vi "Update FOV.vi"(8 "error in (no error)":errorcluster, 11 "UI ctrl refs":T1) -> (0 "error out":errorcluster)   [LabVIEW 2020]
uses:
  Typedefs/UI ctrl refs cluster.ctl
  Typedefs/Laser control knob.ctl
  Typedefs/Frame Size.ctl
  Typedefs/Plane Mode.ctl
  Typedefs/PMT control knob.ctl
  Typedefs/XY Stage_Move.ctl
  Typedefs/test_fpga_control.ctl
  Acquisition/Typedefs/Ref DAQ Param.ctl
  Experiment Type.ctl
  Biology Information.ctl
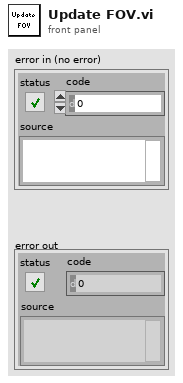
[diagram p1: front panel]
types:
  T1 = typedef "UI ctrl refs cluster.ctl" = cluster{"Top level VI path":path, "Top level VI ref":refnum<vi>, "User menu ref":refnum<k9>, "Sub Panel control":refnum<vi>, "Imaging Param Tab":refnum<vi>, "Occurrence-Start drivers":refnum<k4>, "Occurrence-Speed logging initialised":refnum<k4>, "Occurrence-XYZ stage initialised":refnum<k4>, "Exit button":refnum<vi>, "Status ind":refnum<vi>, "Set as origin":refnum<vi>, "Speed Logging":refnum<vi>, "Time Lapse":refnum<vi>, "Live Imaging":refnum<vi>, "AOL Z Stack":refnum<vi>, "Motor Z Stack":refnum<vi>, "Funct Acq button":refnum<vi>, "Hard Shutter":refnum<vi>, "Virtual Shutter":refnum<vi>, "Laser Power":refnum<vi>, "AOL Mode":refnum<vi>, "Frame Size":refnum<vi>, "Field of View":refnum<vi>, "Dwell Time":refnum<vi>, "Zoom":refnum<vi>, "AOL Z":refnum<vi>, "Objective":refnum<vi>, "Axis":refnum<vi>, "Paths & Names":refnum<vi>, "Experiment folder path (ind.)":refnum<vi>, "Last State (Ind.)":refnum<vi>, "Averages":refnum<vi>, "Angle (degrees)":refnum<vi>, "X centre":refnum<vi>, "Y centre":refnum<vi>, "Plane Mode":refnum<vi>, "# Planes":refnum<vi>, "Z Start":refnum<vi>, "Z Stop":refnum<vi>, "Z Step":refnum<vi>, "PMT 1":refnum<vi>, "PMT 2":refnum<vi>, "Stage XYZ Position":refnum<vi>, "Pockels@Z Start":refnum<vi>, "Pockels@Z Stop":refnum<vi>, "Obtain Z Start":refnum<vi>, "Obtain Z Stop":refnum<vi>, "Live stim.trig.period":refnum<vi>, "Live stim.trig.enable":refnum<vi>, "Movement Correction":refnum<vi>, "Load Reference Image":refnum<vi>, "XY Stage Move":refnum<vi>, "MovCor Cluster":refnum<vi>, "RefDAQParam":refnum<vi>, "Funct. Acq. Pockels Modulation":refnum<vi>, "Ref Laser Power":refnum<vi>, "Enable Video Recording":refnum<vi>, "Video Record-Live Imaging":refnum<vi>, "Video Record-Funct acq":refnum<vi>, "Reference Source":refnum<vi>, "AOL Z-stack Chirps Ready (ind)":refnum<vi>, "Target time between mov.cor. ref triggers (ms)":refnum<vi>, "Funct. Acq. Ref frame save":refnum<vi>, "Tracking button":refnum<vi>, "Show ref plots window":refnum<vi>, "Center freq ind (nm)":refnum<vi>, "Pickup mode (ind)":refnum<vi>, "Logging queue (ind)":refnum<vi>, "Back aperture power (ind.)":refnum<vi>, "Power after objective (ind.)":refnum<vi>, "Switch user":refnum<vi>, "Ls1 Conn. Status":refnum<vi>, "Ls1Tuning Status":refnum<vi>, "Ls1 Faults":refnum<vi>, "Ls1 Connection":refnum<vi>, "Ls1 Mode":refnum<vi>, "Ls1 POWER [mW]":refnum<vi>, "Ls1Shutter":refnum<vi>, "Ls1 Wavelength":refnum<vi>, "Ls1 Note":refnum<vi>, "Ls1 Confirm Wav":refnum<vi>, "Ls1 PreChrp Prism1":refnum<vi>, "Ls1 PreChrp Prism2":refnum<vi>, "Ls1 wav top Ind":refnum<vi>, "Ls1 power top Ind":refnum<vi>, "Ls1 Pump peak Hold":refnum<vi>, "Ls1 Status Ind":refnum<vi>, "Ls1 wav cancel":refnum<vi>, "Experiment Type":refnum<vi>, "Biology Information":refnum<vi>, "Camera recording status":refnum<vi>, "Optimise Obj. Pos.":refnum<vi>}
  T2 = typedef "AOL_Globals.ctl" = cluster{"Imaging Protocol":T3, "Number of POI":u16, "Number of Miniscans":u16, "Number of Trials":u16, "Number of Cycles ":u64, "# Averaged Frames":u16, "Laser power (%)":u8, "Pockels (V)":dbl, "Acquisition Length (sec)":dbl, "Fill time (us)":dbl, "POI Dwell time (us)":dbl, "Miniscan Dwell time per pixel (us)":dbl, "PMT 1":dbl, "PMT 2":dbl, "Back Apperture (mA)":dbl, "Frame Size":T4, "Center Frequency":dbl, "Field of View (um)":dbl, "Field of View (norm)":dbl, "DwellTime (us)":dbl, "Ref Dwell Time (us)":dbl, "Wavelength (nm)":dbl, "Zoom":dbl, "AOL Z":dbl, "AOL Mode":T5, "GridXY":dbl, "GridZ":dbl, "TriggerPeriod (sec)":dbl, "Number of Pixels in Miniscan":u16, "Experiment folder path":path, "X centre":dbl, "Y centre":dbl, "Angle (degrees)":dbl, "Angle Xs (degrees)":dbl, "Angle Ys (degrees)":dbl, "Plane Mode":T6, "Threshold":u16[], "Regenerate Chirps":bool, "Rectangle ROI length (pixels)":u16, "Rectangle ROI height (pixels)":u16, "AOD fill":u16, "StartupDelay":i32, "Samples Wait after Trigger":u16, "Slip Cycle":u32, "Add Cycle":bool, "Functional Mode":T7, "Z Start":dbl, "Z Stop":dbl, "# Planes":i32, "Total Pixels":i32, "Variable Miniscan Pixels":u16[], "Use Variable Length":bool, "Use Variable Resolution":bool, "Laser power (%) at Z Start":u8, "Laser power (%) at Z Stop":u8, "Ref Z Step":i8}
  T3 = typedef "Imaging Protocols enum.ctl" = enum16{"AOL Z-Stack", "Motor Z Stack", "Parameter Sweep", "Functional Acquisition", "Single Plane Acquisition", "Volume Acquisition", "Live Imaging", "Live Plane Imaging", "Live Volume Imaging"}
  T4 = typedef "Frame Size.ctl" = u16
  T5 = typedef "AOL modes.ctl" = enum16{"Raster", "Structural", "Pointing", "Mini Scan", "Alignment"}
  T6 = typedef "Plane Mode.ctl" = u16
  T7 = typedef "Functional Mode.ctl" = enum16{"Point", "Line", "Patch", "Plane", "Volume"}
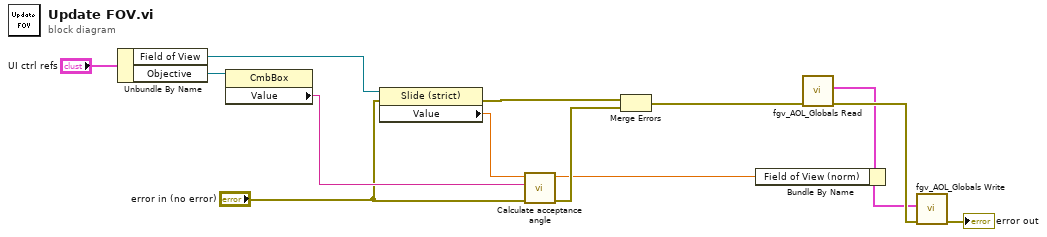
[diagram p0: block diagram]
diagram:
  n1 = Unbundle By Name("UI ctrl refs") -> ("Field of View"=w14:refnum<vi>, "Objective"=w11:refnum<vi>)
  n2 = property on="Property Node" class="CmbBox"(reference=w11) -> ("Value"=w10:string)  [unwired: 1 in, 2 out]
  n3 = property on="Property Node" class="Slide (strict)"(reference=w14, error in="error in (no error)") -> (error out=w7:errorcluster, "Value"=w12:sgl)  [unwired: 1 out]
  n4 = call "Calculate acceptance angle.vi"("error in (no error)"="error in (no error)", "Objective"=w10, "FOV (true)"=w12) -> ("error out"=w8:errorcluster, "Acceptance Angle (mrad)"=w2:dbl)  [unwired: 7 in]
  n5 = Merge Errors(w7, w8) -> (w6:errorcluster)
  n6 = call "fgv_AOL_Globals Read.vi"("error in (no error)"=w6) -> ("error out"=w5:errorcluster, "AOL_Globals"=w4:T2)  [unwired: 8 in, 1 out]
  n7 = Bundle By Name(cluster=w4, "Field of View (norm)"=w2) -> (w3:T2)
  n8 = call "fgv_AOL_Globals Write.vi"("error in (no error)"=w5, "AOL_Globals"=w3) -> ("error out"=→"error out":errorcluster)  [unwired: 9 in]
